vi "reorderSheets.vi"(8 "error in (no error)":errorcluster, 10 "SheetNames":string[](array[string]), 11 "MS-Excel in":refnum<class "MS-Excel.lvclass">) -> (0 "error out":errorcluster, 3 "MS-Excel out":refnum<class "MS-Excel.lvclass">)   [LabVIEW 2017, in "LabVIEW NPOI.lvlib" / "MS-Excel.lvclass"]
uses:
  MS-Excel.lvclass
  D:/Benjamin/Documents/Perso/Code/WC/LabVIEW_NPOI/lib/NPOI 2.1.1/NPOI.dll
  lib/NPOI 2.1.1/NPOI.dll
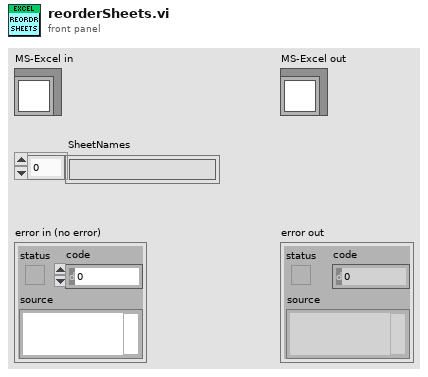
[diagram p1: front panel]
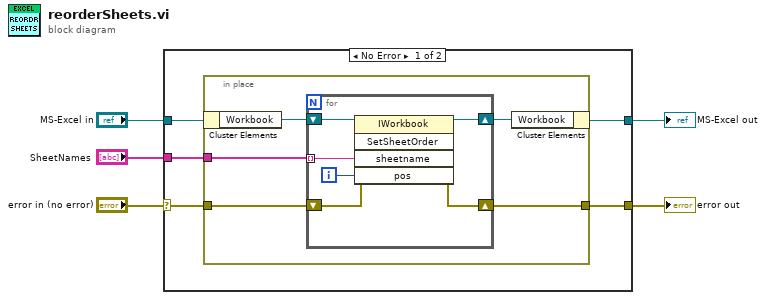
[diagram p0: block diagram]
diagram:
  n1 = case shown="No Error" "error in (no error)" {
    selector: "error in (no error)" -> [w7 w23]
    tunnel: [w6 w23] -> w4
    tunnel: [w9 w22] -> w2
    tunnel: "MS-Excel in" -> [w10 w22]
    tunnel: "SheetNames" -> [w8 _]
    frame No Error {
      n2 = in-place {
        in-place-border: w8 -> [w13]
        in-place-border: w7 -> [w12]
        in-place-border: [w11] -> w6
        n3 = in-place-cluster #1(w10) -> ("Workbook"=w15:refnum<k24>)
        n4 = for {
          shift-right: [w20] -> w14
          shift-left: w15 -> [w21]
          tunnel: w13 -> [w18] mode=indexing
          shift-right: [w16] -> w11
          shift-left: w12 -> [w17]
          i -> [w19]
          n5 = invoke class="IWorkbook" method="SetSheetOrder"(reference=w21, error in=w17, "sheetname"=w18, "pos"=w19) -> (reference out=w20:refnum<k24>, error out=w16:errorcluster)  [unwired: 1 in, 3 out]
        }
        n6 = in-place-cluster #1("Workbook"=w14) -> (w9:refnum<class "MS-Excel.lvclass">)
      }
    }
    frame Error {
    }
  }
  "error out" <- w4
  "MS-Excel out" <- w2
